vi "Read Manual Range.vi"(8 "error in (no error)":errorcluster, 11 "34401 in":refnum<class "34401.lvclass">) -> (0 "error out":errorcluster, 2 "Manual Range":dbl=1.0, 3 "34401 out":refnum<class "34401.lvclass">)   [LabVIEW 2018, in "34401.lvlib" / "34401.lvclass"]
uses:
  34401.lvclass
  34401.lvclass/34401.ctl
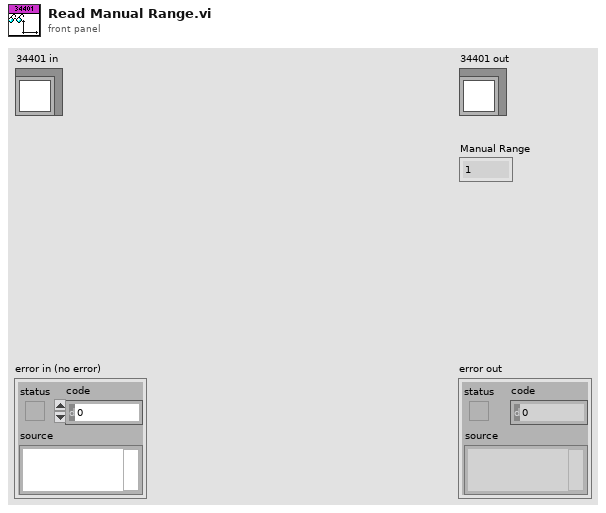
[diagram p1: front panel]
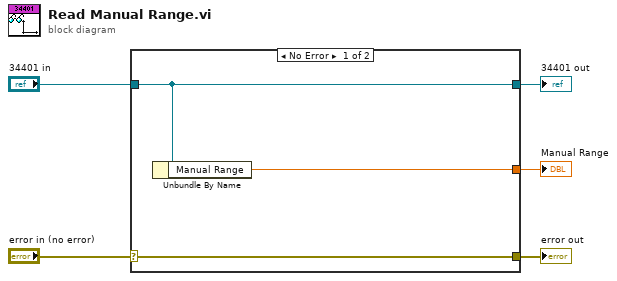
[diagram p0: block diagram]
diagram:
  n1 = case shown="No Error" "error in (no error)" {
    selector: "error in (no error)" -> [w8 w9]
    tunnel: [w8 w9] -> w4
    tunnel: [w7 w10] -> w2
    tunnel: "34401 in" -> [w7 w10]
    tunnel: [w6 _] -> w1
    frame No Error {
      n2 = Unbundle By Name(w7) -> ("Manual Range"=w6:dbl)
    }
    frame Error {
    }
  }
  "error out" <- w4
  "34401 out" <- w2
  "Manual Range" <- w1
